vi "EMBALLAGE_BDD_ZebraPrinter_IPComplet.vi"(1 "Liste IP":string[](array[string]), 2 "indice":i32) -> (0 "IP Zebra complet":string)   [LabVIEW 2020]
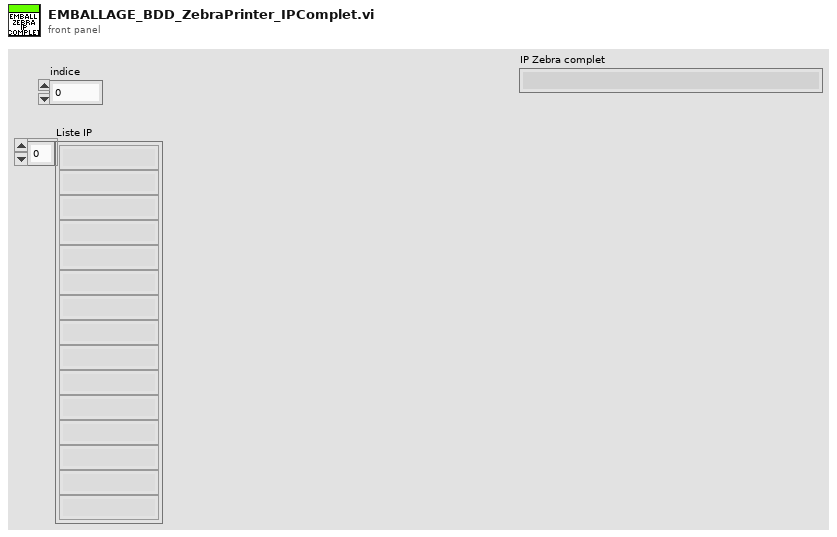
[diagram p1: front panel]
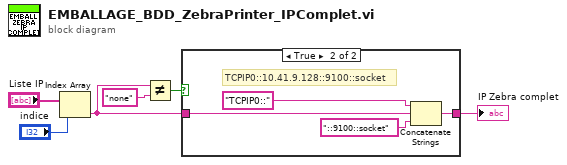
[diagram p0: block diagram]
diagram:
  n1 = Index Array(array="Liste IP", index="indice") -> (element=w3:string)
  n2 = Not Equal?(x=w3, y="none") -> (x != y?=w2:bool)
  n3 = case shown="True" w2 {
    tunnel: [w7 w11] -> w5
    tunnel: w3 -> [w7 w10]
    frame False {
    }
    frame True {
      # "TCPIP0::10.41.9.128::9100::socket"
      n4 = Concatenate Strings("TCPIP0::", w10, "::9100::socket") -> (w11:string)
    }
  }
  "IP Zebra complet" <- w5
